vi "Select_USB_CAN_Device.vi"(11 "DevNames":string[](array[string])) -> (3 "DevNum":i32)   [LabVIEW 2011]
panel:
  in  "cancel":bool
  in  "ok":bool
  in  "DeviceName":i32(ring) caption="设备名称：" items=["0229", "0299", "0300"]
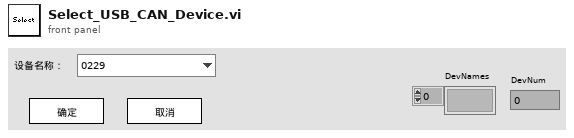
[diagram p1: front panel]
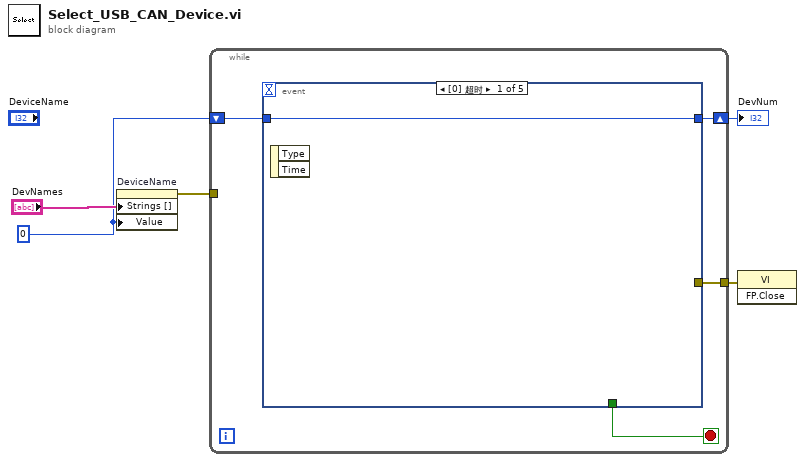
[diagram p0: block diagram]
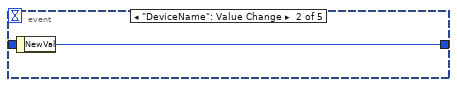
[diagram p2: hidden frame]
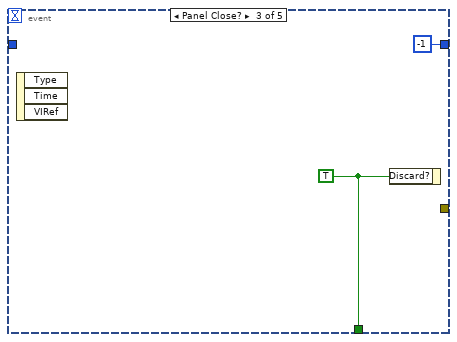
[diagram p3: hidden frame]
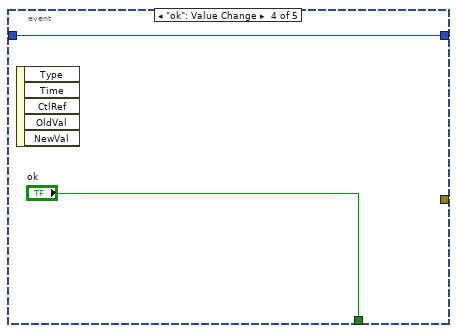
[diagram p4: hidden frame]
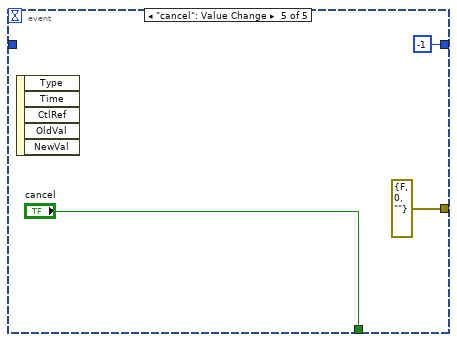
[diagram p5: hidden frame]
diagram:
  w1 = 0
  n1 = property on="DeviceName" class="Ring (严格)"("Strings []"="DevNames", "Value"=w1) -> (error out=w4:errorcluster)  [unwired: 2 in, 1 out]
  n2 = while {
    tunnel: w4 -> [_]
    shift-right: [w7] -> w3
    shift-left: w1 -> [w8]
    tunnel: [w6] -> w2
    stop <- w9 stop-if-true
    n3 = event shown="[0] 超时" {
      selector: _ -> [_ _ _ _ _]
      dyn-events: _ -> [_ _ _ _ _]
      timeout: _ -> [_ _ _ _ _]
      tunnel: [_ _ w13 "ok" "cancel"] -> w9
      tunnel: w8 -> [w10 _ _ w14 _]
      tunnel: [w10 w11 -1 ("DeviceName") w14 -1 ("DeviceName")] -> w7
      tunnel: [_ _ _ _ errorcluster {"status"=FALSE, "code"=0, "source"=""} ("错误输入（无错误）")] -> w6
      event Timeout {
        n4 = event-data() -> ()  [unwired: 1 in, 2 out]
      }
      event "DeviceName": Value Change {
        n5 = event-data() -> ("NewVal"=w11:i32)  [unwired: 1 in]
      }
      event Panel Close? {
        w13 = TRUE ("放弃？")
        n6 = event-data() -> ()  [unwired: 1 in, 3 out]
        n7 = event-data("Discard?"=w13) -> ()  [unwired: 1 in, 1 out]
      }
      event "ok": Value Change {
        n8 = event-data() -> ()  [unwired: 1 in, 5 out]
      }
      event "cancel": Value Change {
        n9 = event-data() -> ()  [unwired: 1 in, 5 out]
      }
    }
  }
  "DevNum" <- w3
  n10 = invoke class="VI" method="FP.Close"(error in=w2) -> ()  [unwired: 2 in, 3 out]
